vi "Matlab_SimplePlot.vi"() -> ()   [LabVIEW 2018]
uses:
  <vilib>/Utility/error.llb/Error Cluster From Error Code.vi
  <vilib>/ErrorRing/Error Ring.xnode
panel:
  out "Error Out":errorcluster
  out "Data (In)":dbl[][](array[numeric])
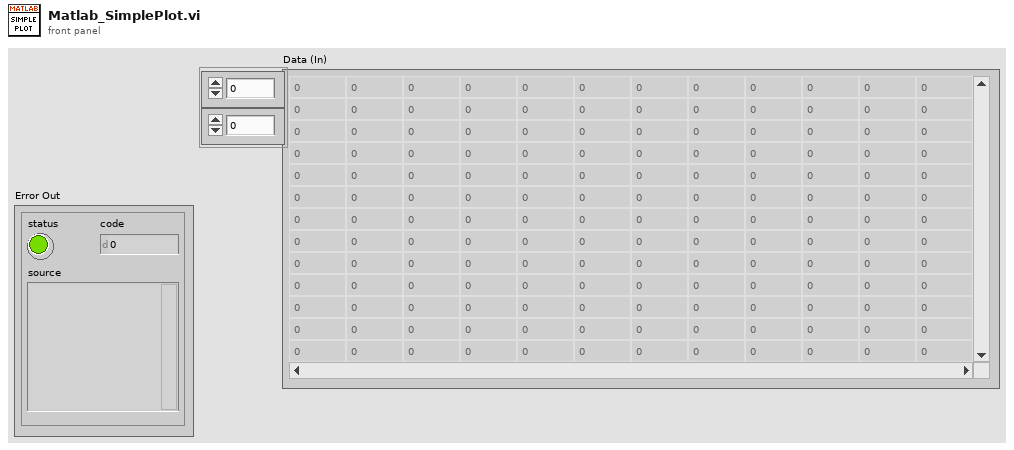
[diagram p1: front panel]
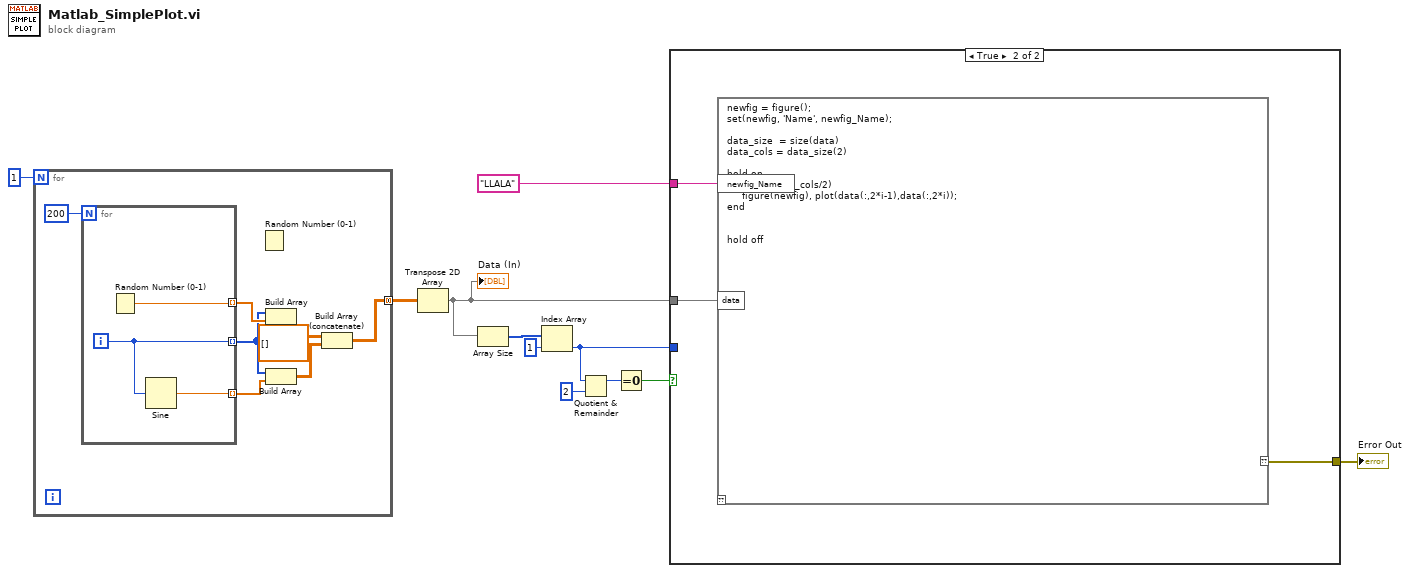
[diagram p0: block diagram]
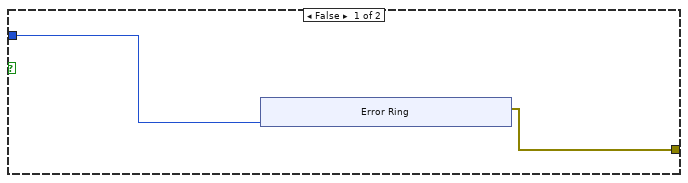
[diagram p2: hidden frame]
diagram:
  n1 = for {
    N: 1 -> [_]
    tunnel: [w13] -> w10 mode=concatenating
    n2 = for {
      N: 200 -> [_]
      tunnel: [w21] -> w17 mode=indexing
      tunnel: [w20] -> w16 mode=indexing
      tunnel: [w19] -> w15 mode=indexing
      i -> [w20]
      n3 = Random Number (0-1)() -> (number: 0 to 1=w21:dbl)
      n4 = Sine(x=w20) -> (sin(x)=w19:dbl)
    }
    n5 = Random Number (0-1)() -> ()  [unwired: 1 out]
    n6 = Build Array(w16, w17) -> ()  [unwired: 1 out]
    n7 = Build Array(w16, w15) -> (w14:dbl[][])
    n8 = Build Array (concatenate)(dbl[][] [] ("array"), w14) -> (w13:dbl[][])
  }
  n9 = Transpose 2D Array(2D array=w10) -> (transposed array=w7:dbl[][])
  "Data (In)" <- w7
  n10 = Array Size(array=w7) -> (size(s)=w6:i32[])
  n11 = Index Array(array=w6, index=1) -> (element=w1:i32)
  n12 = Quotient & Remainder(x=w1, y=2 ("index")) -> (x-y*floor(x/y)=w3:i32)  [unwired: 1 out]
  n13 = Equal To 0?(x=w3) -> (x = 0?=w2:bool)
  n14 = case shown="True" w2 {
    tunnel: "LLALA" -> [_ w33]
    tunnel: [w23 w32] -> w8
    tunnel: w7 -> [_ w31]
    tunnel: w1 -> [w22 _]
    frame False {
      n15 = xnode "Error Ring"("parameter 0"=w22) -> ("error out"=w23:errorcluster)
    }
    frame True {
      n16 = script code="newfig = figure();\nset(newfig, 'Name', newfig_Name);\n\ndata_size  = size(data)\ndata_cols = data_size(2)\n\nhold on\nfor i = 1:(data_cols/2)\n     figure(newfig), plot(data(:,2*i-1),data(:,2*i));\nend\n\n\nhold off"("data"=w31, "newfig_Name"=w33) -> ("??"=w32:errorcluster)  [unwired: 1 in]
    }
  }
  "Error Out" <- w8
